vi "Read Max Amps.vi"(8 "error in (no error)":errorcluster, 11 "Keithley230X-Fix in":refnum<class "Keithley230X-Fix.lvclass">) -> (0 "error out":errorcluster, 2 "Max Amps":dbl, 3 "Keithley230X-Fix out":refnum<class "Keithley230X-Fix.lvclass">)   [LabVIEW 2020, in "LAF2024Q2.lvlib" / "Keithley230X-Fix.lvclass"]
uses:
  Keithley230X-Fix.lvclass
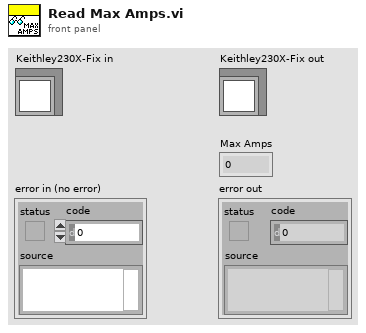
[diagram p1: front panel]
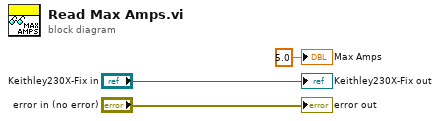
[diagram p0: block diagram]
diagram:
  "error out" <- "error in (no error)"
  "Keithley230X-Fix out" <- "Keithley230X-Fix in"
  "Max Amps" <- 5.0 ("Max Amps")
